vi "File Logging - Fire Event.vi"() -> ()   [LabVIEW 2009]
uses:
  Controls/SLL DE DO Command LV2Global Options.ctl
  Controls/SLL DE File Logging Command List.ctl
panel:
  out "Error out":errorcluster
  in  "Option 2":T1=enum."Stop Logging"
  in  "Option":T2=enum."Fire Event"
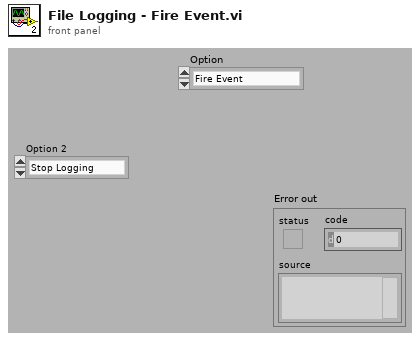
[diagram p1: front panel]
types:
  T1 = typedef "SLL DE File Logging Command List.ctl" = enum16{"Start Logging", "Stop Logging"}
  T2 = typedef "SLL DE DO Command LV2Global Options.ctl" = enum16{"Init/Register Events", "Get Event Refnum", "Fire Event", "Distroy Event"}
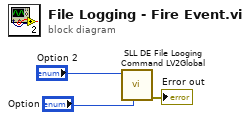
[diagram p0: block diagram]
diagram:
  n1 = call "SLL DE File Looging Command LV2Global.vi"("Option"="Option", "File Logging Option"="Option 2") -> ("Error out"=→"Error out":errorcluster)  [unwired: 1 in, 8 out]
